vi "demo_hub.vi"() -> ()   [LabVIEW 2017]
panel:
  in  "ip":string="192.168.1.44"
  out "数字":i32 format="%x"
  in  "name":string="hub1"
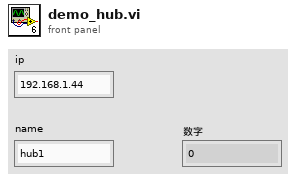
[diagram p1: front panel]
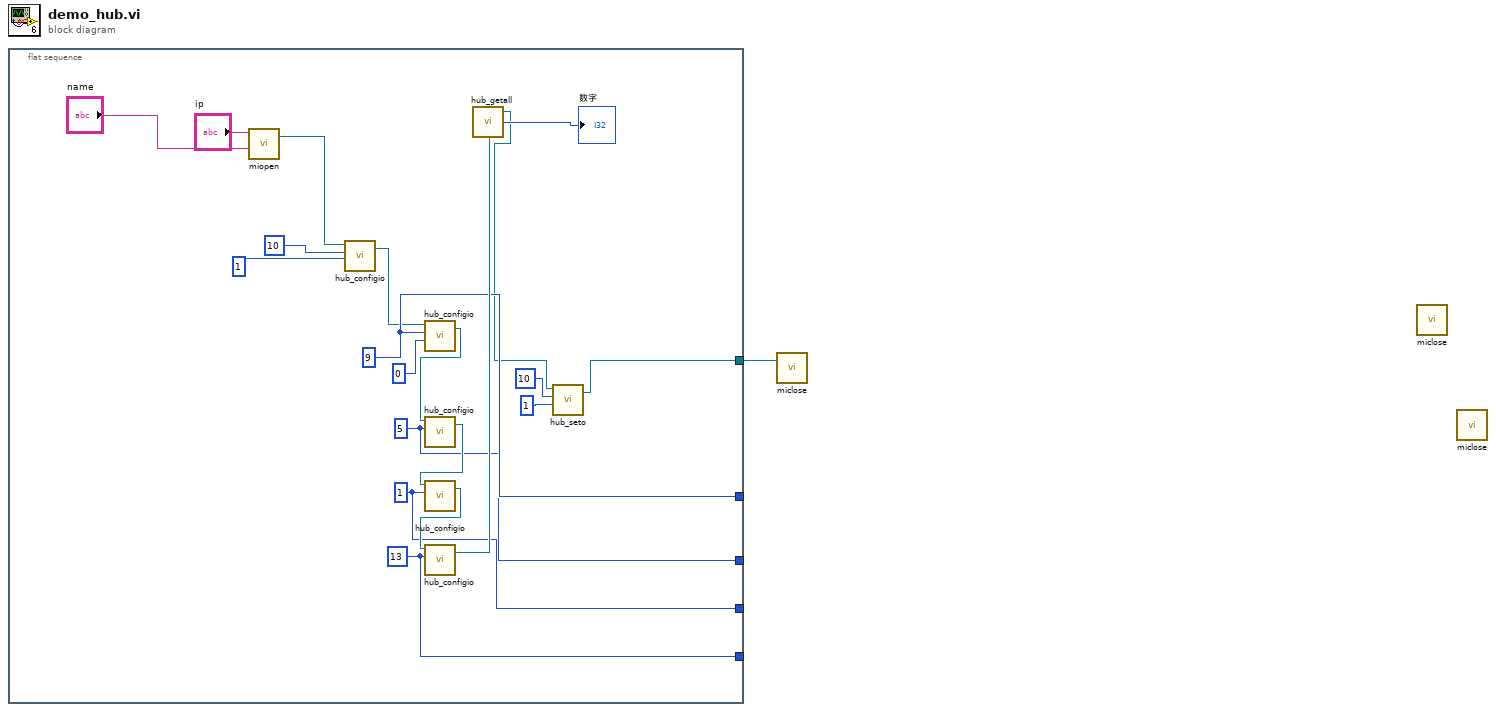
[diagram p0: block diagram]
diagram:
  n1 = flat-sequence {
    tunnel: [w4] -> w1
    tunnel: [w14] -> _
    tunnel: [w13] -> _
    tunnel: [w12] -> _
    tunnel: [w11] -> _
    frame #0 {
      w11 = 13 ("输入 1")
      w12 = 1 ("输入 1")
      w13 = 5 ("输入 1")
      w14 = 9 ("输入 1")
      n2 = call "miopen.vi"("name"="name", "ip"="ip") -> ("VISA资源名称输出"=w9:refnum<visa-resource-name>)  [unwired: 2 in, 1 out]
      n3 = call "hub_configio.vi"("输入 2"=1, "输入 1"=10, "VISA资源名称"=w9) -> ("VISA资源名称输出"=w8:refnum<visa-resource-name>)  [unwired: 1 in, 1 out]
      n4 = call "hub_configio.vi"("输入 2"=0, "输入 1"=w14, "VISA资源名称"=w8) -> ("VISA资源名称输出"=w19:refnum<visa-resource-name>)  [unwired: 1 in, 1 out]
      n5 = call "hub_configio.vi"("输入 1"=w13, "VISA资源名称"=w19) -> ("VISA资源名称输出"=w18:refnum<visa-resource-name>)  [unwired: 2 in, 1 out]
      n6 = call "hub_configio.vi"("输入 1"=w12, "VISA资源名称"=w18) -> ("VISA资源名称输出"=w17:refnum<visa-resource-name>)  [unwired: 2 in, 1 out]
      n7 = call "hub_configio.vi"("输入 1"=w11, "VISA资源名称"=w17) -> ("VISA资源名称输出"=w16:refnum<visa-resource-name>)  [unwired: 2 in, 1 out]
      n8 = call "hub_getall.vi"("VISA资源名称"=w16) -> ("VISA资源名称输出"=w5:refnum<visa-resource-name>, "数字"=→"数字":i32)  [unwired: 1 in, 1 out]
      n9 = call "hub_seto.vi"("输入 2"=1, "输入 1"=10, "VISA资源名称"=w5) -> ("VISA资源名称输出"=w4:refnum<visa-resource-name>)  [unwired: 1 in, 1 out]
    }
  }
  n10 = call "miclose.vi"("VISA资源名称"=w1) -> ()  [unwired: 1 in, 1 out]
  n11 = call "miclose.vi"() -> ()  [unwired: 2 in, 1 out]
  n12 = call "miclose.vi"() -> ()  [unwired: 2 in, 1 out]
